vi "SendNested.vi"(8 "error in (no error)":errorcluster, 10 "Message":string, 11 "Caller in":refnum<class "Caller.lvclass">) -> (0 "error out":errorcluster, 3 "Caller out":refnum<class "Caller.lvclass">)   [LabVIEW 2020, in "Caller.lvlib" / "Caller.lvclass"]
uses:
  Caller.lvclass
  Caller.lvclass/Caller.ctl
  Nested Messages/UpdateDIsplayNested Msg/UpdateDIsplayNested Msg.lvclass/UpdateDIsplayNested Msg.ctl
  <vilib>/ActorFramework/Message Enqueuer/Message Enqueuer.lvclass/Message Enqueuer.ctl
  <vilib>/ActorFramework/Message Enqueuer/Enqueue.vi
  Nested Messages/UpdateDIsplayNested Msg/UpdateDIsplayNested Msg.lvclass
  C:/Program Files/National Instruments/LabVIEW 2020/vi.lib/ActorFramework/Message/Message.lvclass
  <vilib>/ActorFramework/Message Priority Queue/Priority Enqueue.vi
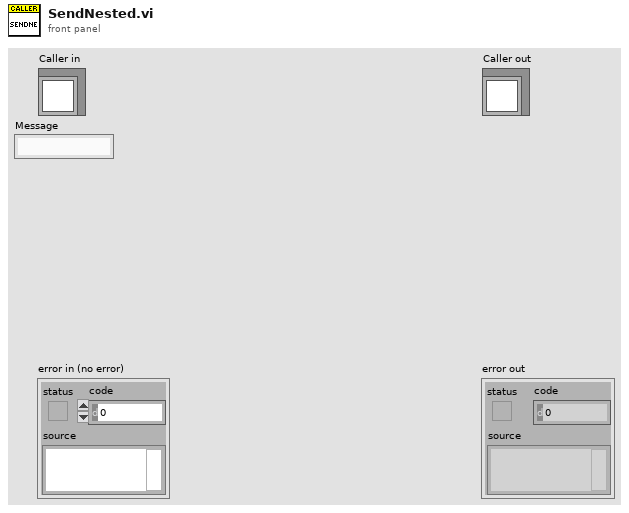
[diagram p1: front panel]
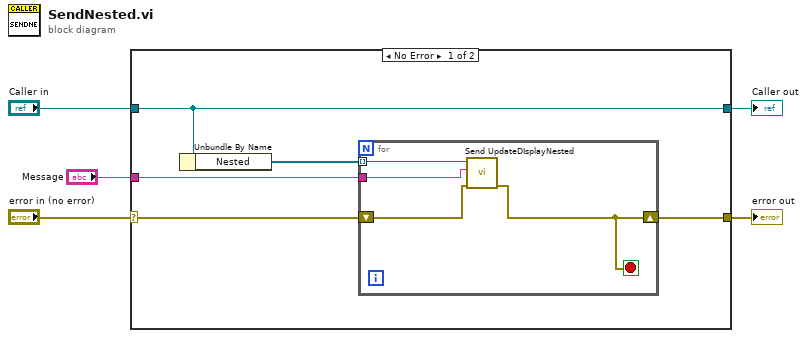
[diagram p0: block diagram]
diagram:
  n1 = case shown="No Error" "error in (no error)" {
    selector: "error in (no error)" -> [w7 w16]
    tunnel: [w6 w16] -> w4
    tunnel: [w10 w15] -> w2
    tunnel: "Caller in" -> [w10 w15]
    tunnel: "Message" -> [w8 _]
    frame No Error {
      n2 = Unbundle By Name(w10) -> ("Nested"=w9:refnum<class "Message Enqueuer.lvclass">[])
      n3 = for {
        tunnel: w9 -> [w14] mode=indexing
        tunnel: w8 -> [w13]
        shift-right: [w11] -> w6
        shift-left: w7 -> [w12]
        stop <- w11 stop-if-true
        n4 = call "Send UpdateDIsplayNested.vi"("error in (no error)"=w12, "Message"=w13, "Message Enqueuer"=w14) -> ("error out"=w11:errorcluster)  [unwired: 7 in, 1 out]
      }
    }
    frame Error {
    }
  }
  "error out" <- w4
  "Caller out" <- w2
